vi "GPIOs.vi"(8 "error in (no error)":errorcluster, 11 "UART in":refnum<class "UART.lvclass">) -> (0 "error out":errorcluster, 1 "RX GPIO":T1, 2 "TX GPIO":T1, 3 "UART out":refnum<class "UART.lvclass">)   [LabVIEW 2020, in "CTI.lvlib" / "UART.lvclass"]
uses:
  UART.lvclass
  GPIO Number.ctl
  UART.lvclass/UART.ctl
  CTI.lvlib
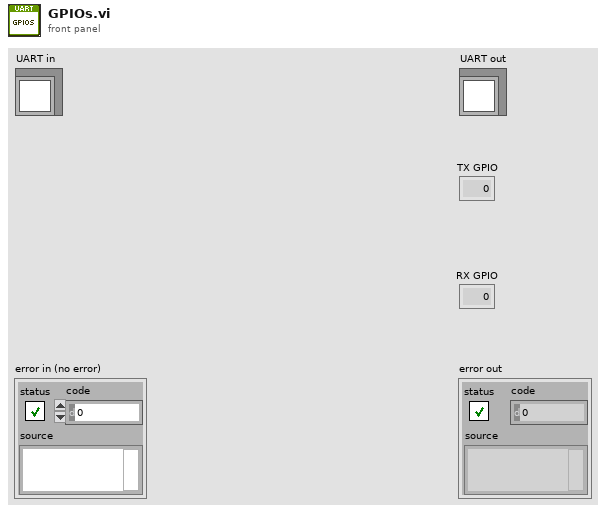
[diagram p1: front panel]
types:
  T1 = typedef "CTI.lvlib/GPIO Number.ctl" = i8
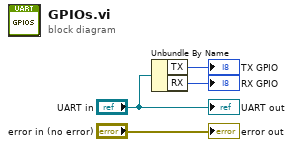
[diagram p0: block diagram]
diagram:
  n1 = Unbundle By Name("UART in") -> ("TX"=→"TX GPIO":T1, "RX"=→"RX GPIO":T1)
  "error out" <- "error in (no error)"
  "UART out" <- "UART in"
